vi "TestLoop_GetClassName.vi"() -> ()   [LabVIEW 2017, in "TestLibrary.lvlib"]
uses:
  TestLibrary.lvlib
panel:
  out "x-y":dbl
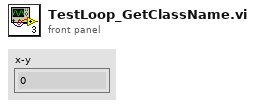
[diagram p1: front panel]
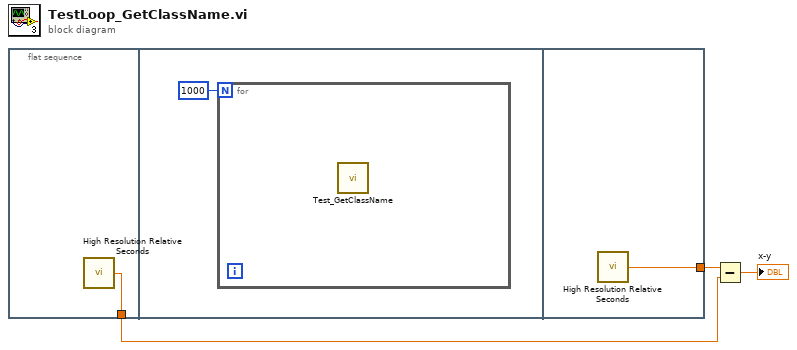
[diagram p0: block diagram]
diagram:
  n1 = flat-sequence {
    tunnel: [w4] -> w2
    tunnel: [w6] -> w3
    frame #0 {
      n2 = call <vilib>:"High Resolution Relative Seconds.vi"() -> ("relative seconds"=w4:dbl)
    }
    frame #1 {
      n3 = for {
        N: 1000 -> [_]
        n4 = call "Test_GetClassName.vi"() -> ()  [unwired: 20 in]
      }
    }
    frame #2 {
      n5 = call <vilib>:"High Resolution Relative Seconds.vi"() -> ("relative seconds"=w6:dbl)
    }
  }
  n6 = Subtract(x=w3, y=w2) -> (x-y=→"x-y":dbl)
